vi "Read ADC Conversion Settings.vi"(11 "ILC in":refnum<class "ILC.lvclass">) -> (2 "ADC Conversion Settings":T1={"Reference Voltage Vref"=0.0, "Nominal Input Range in Counts"=128, "Preamplifier Gain (K1 * K2)"=0.0, "Conversion Settling Cycles"=0, "Excitation Voltage Vexc"=0.0} {"Excitation Voltage Vexc" min=-10.0 max=10.0 format="%.3f"; "Conversion Settling Cycles" min=1; "Preamplifier Gain (K1 * K2)" min=1.0 format="%.2f"; "Nominal Input Range in Counts" min=128; "Reference Voltage Vref" min=-10.0 max=10.0 format="%.3f"}, 3 "ILC out":refnum<class "ILC.lvclass">)   [LabVIEW 2015, in "ILCCommon.lvlib" / "ILC.lvclass"]
uses:
  <userlib>/Common/ILC/ILC/ILC.lvclass
  <userlib>/Common/ILC/Configuration/ADC Conversion Settings.ctl
  <userlib>/Common/ILC/ILC/ILC.lvclass/ILC.ctl
  <userlib>/Common/ILC/Configuration/ILCConfiguration.lvlib
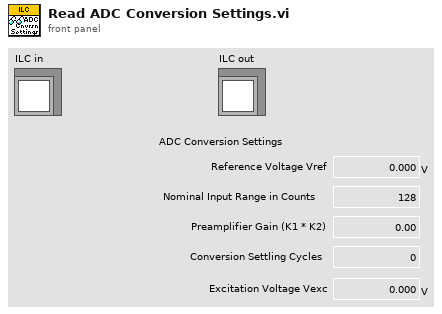
[diagram p1: front panel]
types:
  T1 = typedef "ILCCommon.lvlib/ILCConfiguration.lvlib/ADC Conversion Settings.ctl" = cluster{"Reference Voltage Vref":dbl[unit], "Nominal Input Range in Counts":u32, "Preamplifier Gain (K1 * K2)":dbl, "Conversion Settling Cycles":u16, "Excitation Voltage Vexc":dbl[unit]}
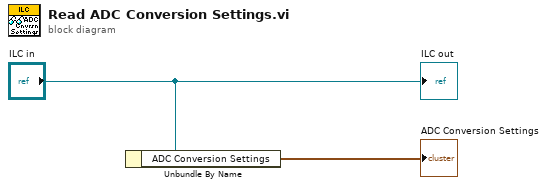
[diagram p0: block diagram]
diagram:
  n1 = Unbundle By Name("ILC in") -> ("ADC Conversion Settings"=→"ADC Conversion Settings":T1)
  "ILC out" <- "ILC in"
